vi "Tray_TraySetPanel.vi"(8 "error in":errorcluster, 11 "Enum_TrayType":T1) -> (0 "error Out":errorcluster)   [LabVIEW 2015]
uses:
  subvi/Tray/Tray_TrayName.ctl
  <vilib>/Utility/miscctls.llb/LVPointTypeDef.ctl
  subvi/Tray/Tray_TrayCtrl_Action.ctl
  LLB/Message/Ctrl/MsgDataInput.ctl
  LLB/Message/Ctrl/MsgPageSelect.ctl
  LLB/Message/Ctrl/MsgTyp.ctl
  LLB/Message/Ctrl/LogType.ctl
  global/Tray_ArrAndData.vi
  LLB/Message/MsgShowAndLog.lvlib
panel:
  out "Flg_Edit":bool
  out "TrayItemStatus":bool[][](array[boolean])
  out "Tray":cluster{"X":i32, "Y":i32}
  in  "Btn_Ini":bool
  in  "Set":bool
  in  "ItemExist":u32(colorbox)=16860
  in  "NoItem":u32(colorbox)=11121611
  in  "SingleSet":bool caption="SetType"
  in  "StatusArr":bool[][](array[boolean])
  in  "Stop Button":bool
  in  "BtnArr":bool[][](array[boolean])
  out "TrayIn":cluster{"Color":u32[][], "Data":string[][]}={"Color"=[[16860, 16860, 16860, 16860, 16860, 16860, 16860, 16860], [16860, 16860, 16860, 16860, 16860, 16860, 16860, 16860], [16860, 16860, 16860, 16860, 16860, 16860, 16860, 16860], [16860, 16860, 16860, 16860, 16860, 16860, 16860, 16860], [16860, 16860, 16860, 16860, 16860, 16860, 16860, 16860], [16860, 16860, 16860, 16860, 16860, 16860, 16860, 16860], [16860, 16860, 16860, 16860, 16860, 16860, 16860, 16860], [16860, 16860, 16860, 16860, 16860, 16860, 16860, 16860], [16860, 16860, 16860, 16860, 16860, 16860, 16860, 16860], [16860, 16860, 16860, 16860, 16860, 16860, 16860, 16860], [16860, 16860, 16860, 16860, 16860, 16860, 16860, 16860], [16860, 16860, 16860, 16860, 16860, 16860, 16860, 16860]], "Data"=[["", "", "", "", "", "", "", ""], ["", "", "", "", "", "", "", ""], ["", "", "", "", "", "", "", ""], ["", "", "", "", "", "", "", ""], ["", "", "", "", "", "", "", ""], ["", "", "", "", "", "", "", ""], ["", "", "", "", "", "", "", ""], ["", "", "", "", "", "", "", ""], ["", "", "", "", "", "", "", ""], ["", "", "", "", "", "", "", ""], ["", "", "", "", "", "", "", ""], ["", "", "", "", "", "", "", ""]]}
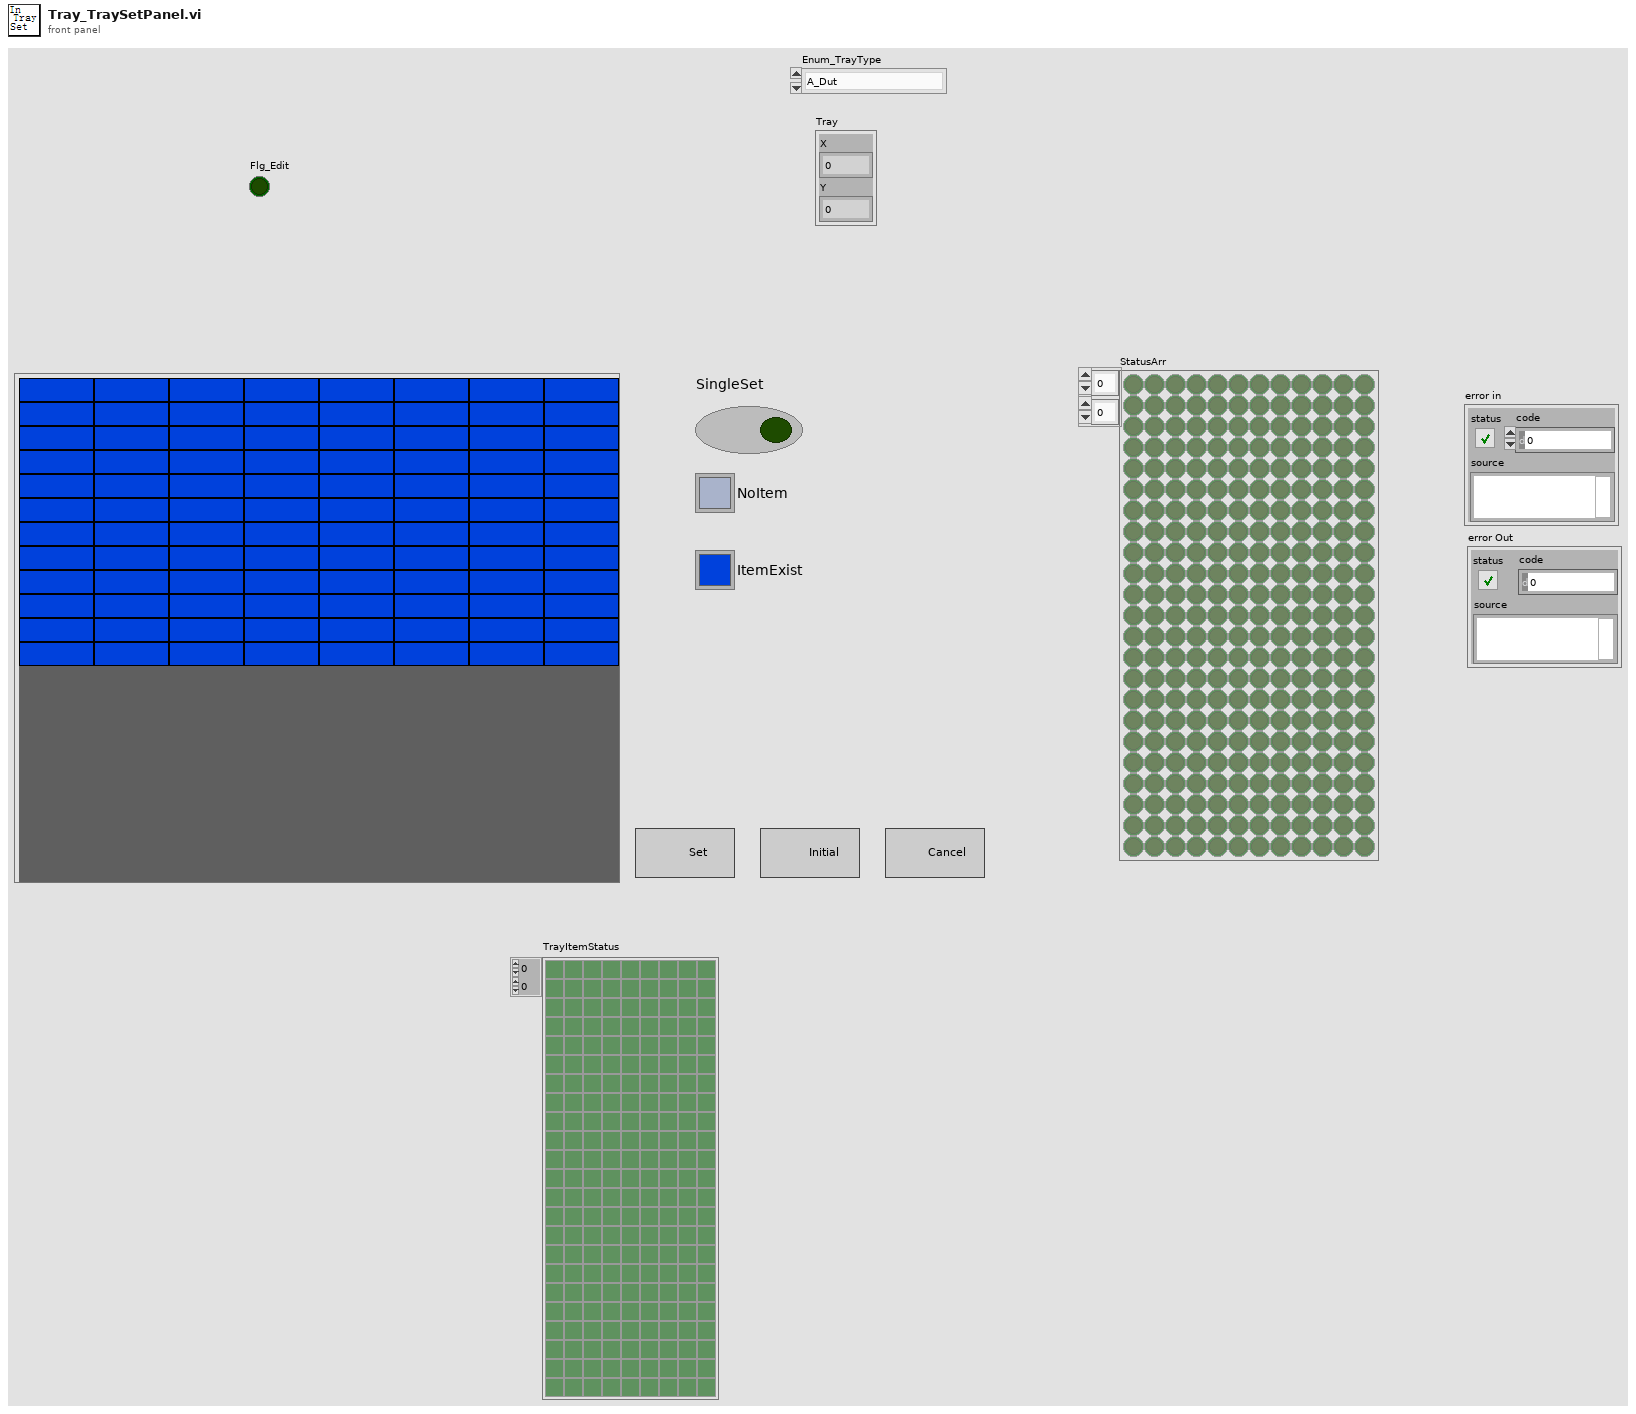
[diagram p1: front panel]
types:
  T1 = typedef "Tray_TrayName.ctl" = enum16{"A_Dut", "B_Pass", "C_NGR", "D_NGL"}
  T2 = typedef "LVPointTypeDef.ctl" = cluster{"Horizontal":i16, "Vertical":i16}
  T3 = cluster{"BtnArr":refnum<vi>, "BtnRef":refnum<vi>}
  T4 = typedef "MsgDataInput.ctl" = cluster{"MsgPageSelect":T5, "Type":T6, "LogType":T7, "Msg":string, "Time":string}
  T5 = typedef "MsgShowAndLog.lvlib/MsgPageSelect.ctl" = enum16{"System", "Robot", "IO", "CCD", "Action", "Alarm", "ATS"}
  T6 = typedef "MsgShowAndLog.lvlib/MsgTyp.ctl" = enum16{"SYS", "TCP/IP", "IO", "CCD", "Action", "RS232"}
  T7 = typedef "MsgShowAndLog.lvlib/LogType.ctl" = enum16{"AutoRun", "Manual", "Error", "ATS"}
  T8 = typedef "Tray_TrayCtrl_Action.ctl" = enum16{"InitialTray", "TrayOut", "TrayIn", "SetTray", "TrayDataToUI"}
  T9 = cluster{"XY_ATray":cluster{"X":i32, "Y":i32}, "Initial color":u32, "FinalColor":u32}
  T10 = cluster{"XY_BTray":cluster{"X":i32, "Y":i32}, "Initial color":u32, "FinalColor":u32}
  T11 = cluster{"XY_CTray":cluster{"X":i32, "Y":i32}, "Initial color":u32, "FinalColor":u32}
  T12 = cluster{"XY_DTray":cluster{"X":i32, "Y":i32}, "Initial color":u32, "FinalColor":u32}
  T13 = typedef "LVPositionTypeDef.ctl" = cluster{"Left":i32, "Top":i32}
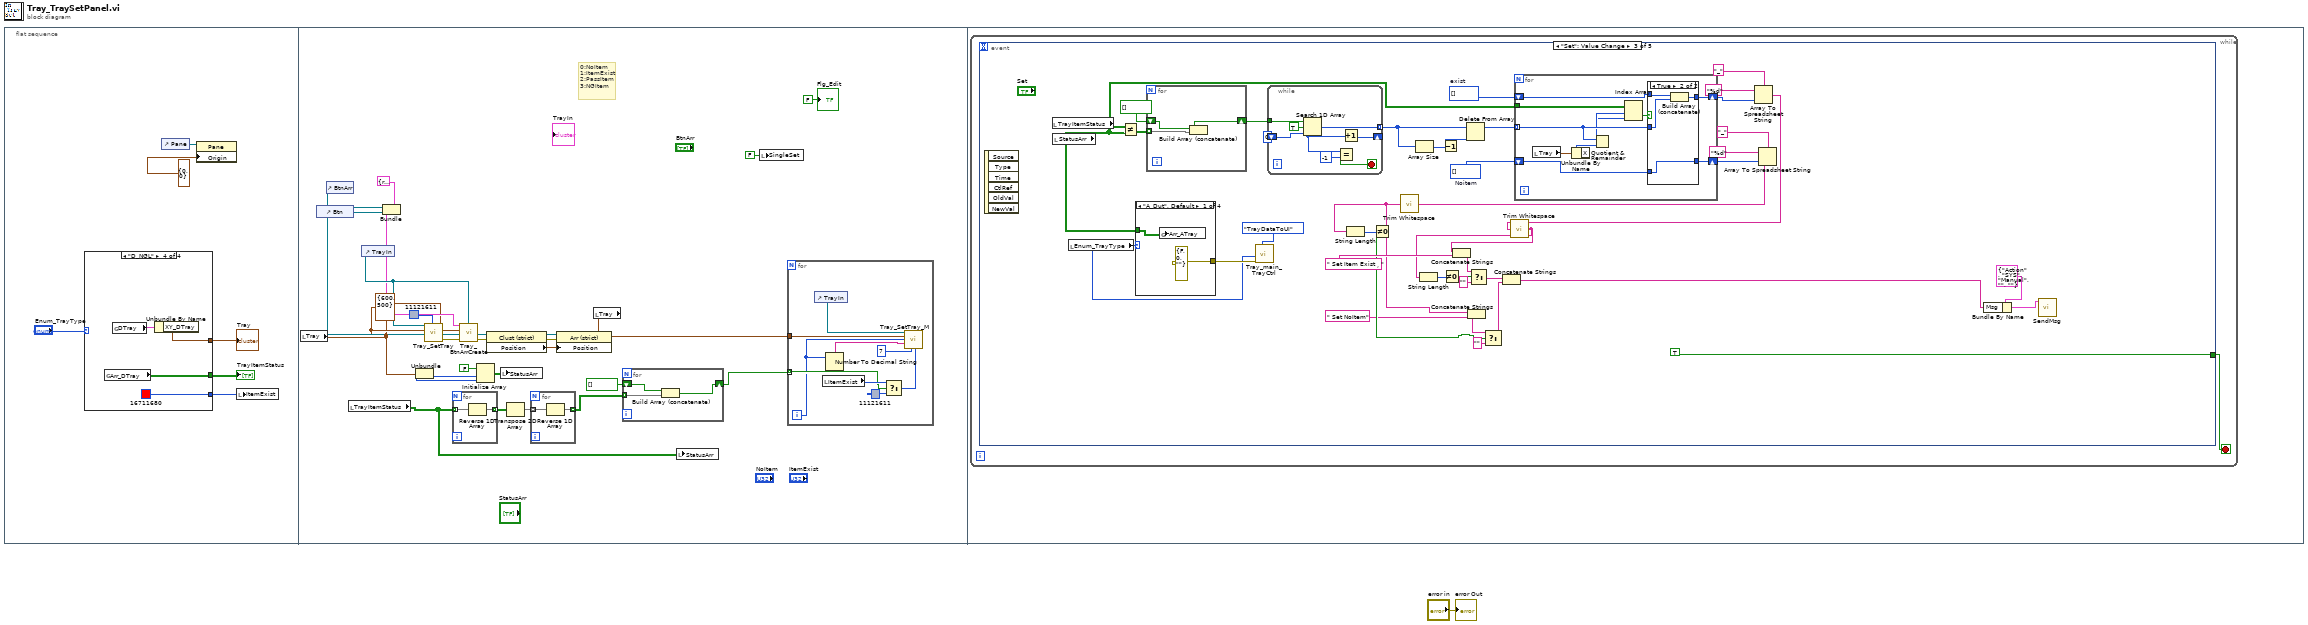
[diagram p0: block diagram]
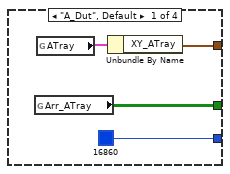
[diagram p2: hidden frame]
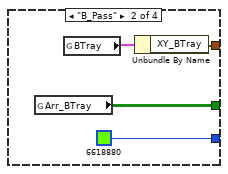
[diagram p3: hidden frame]
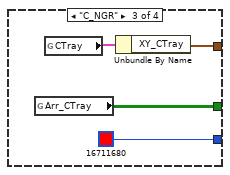
[diagram p4: hidden frame]
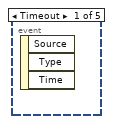
[diagram p5: hidden frame]
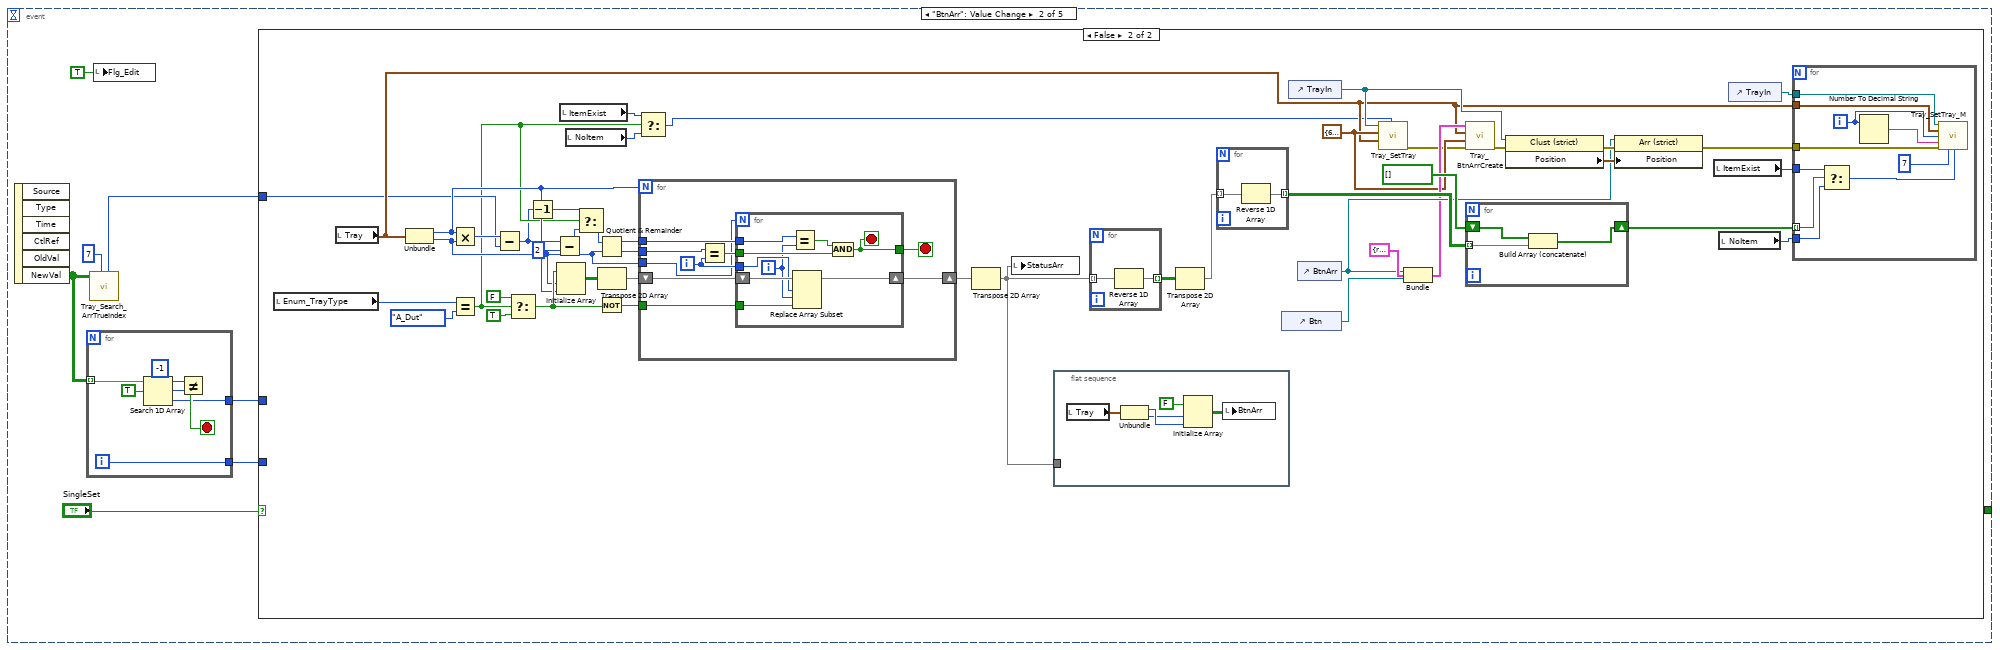
[diagram p6: hidden frame]
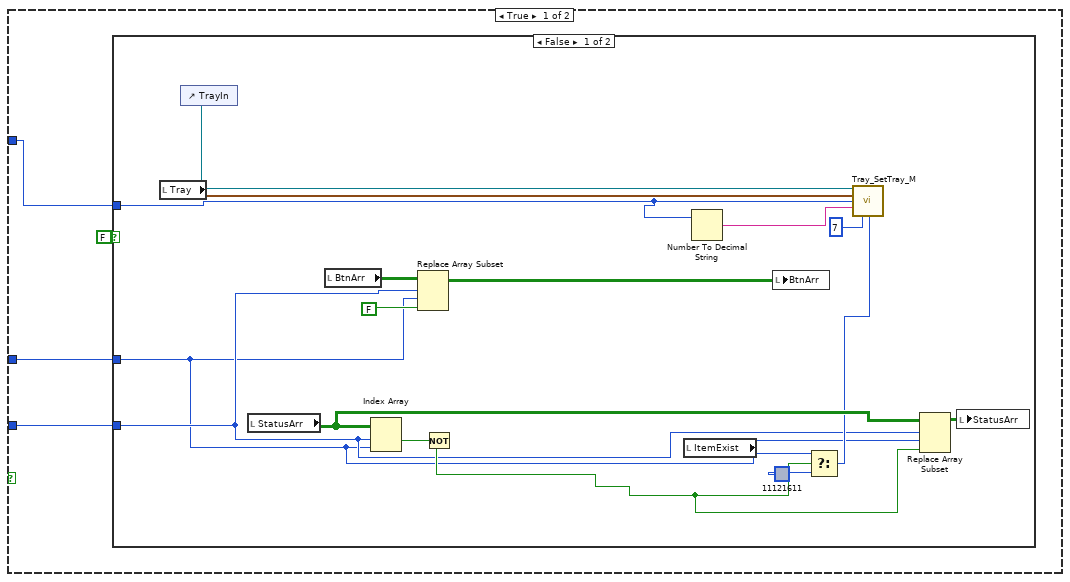
[diagram p7: hidden frame]
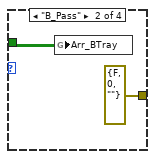
[diagram p9: hidden frame]
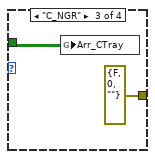
[diagram p10: hidden frame]
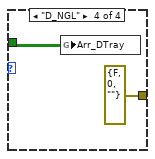
[diagram p11: hidden frame]
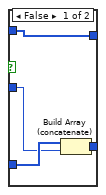
[diagram p12: hidden frame]
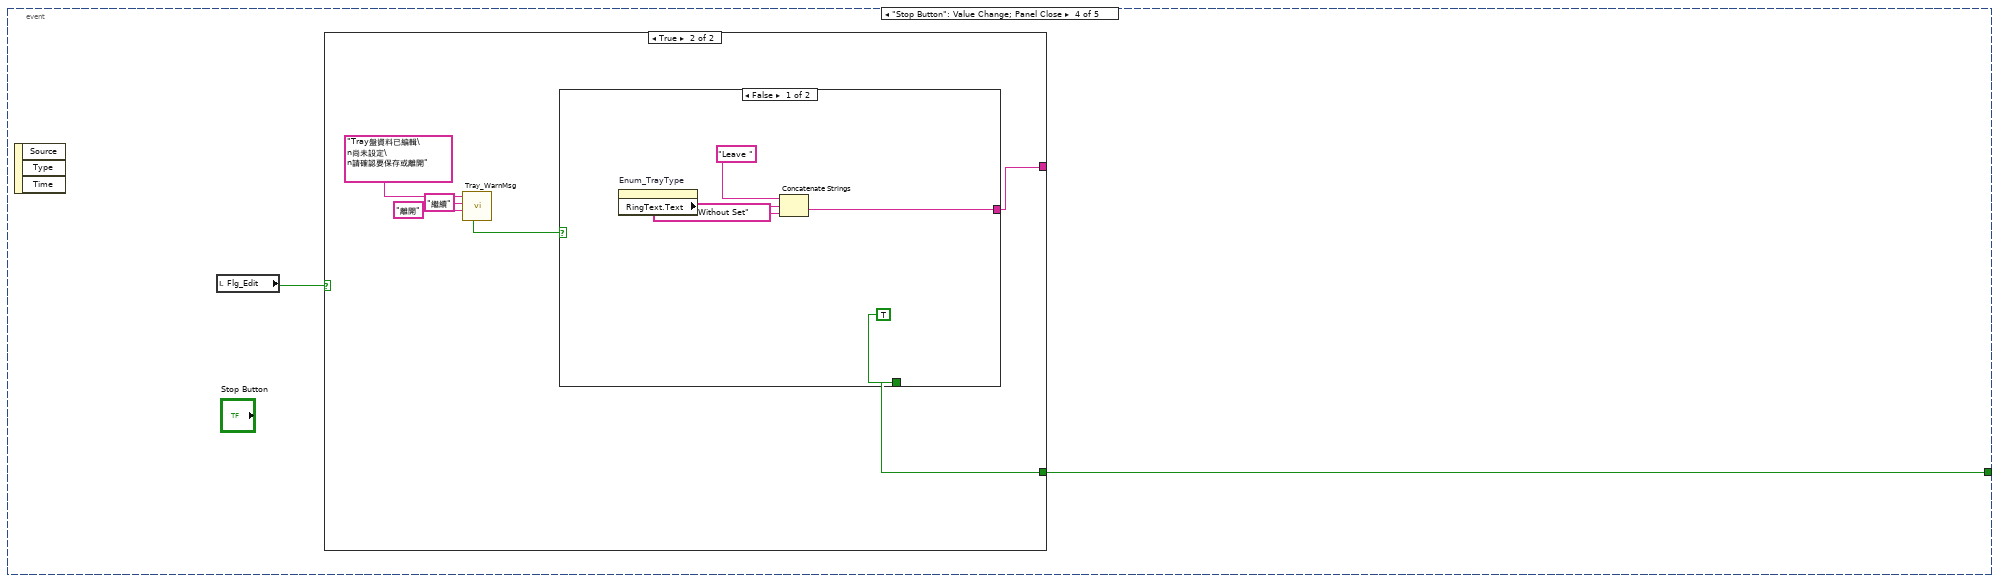
[diagram p13: hidden frame]
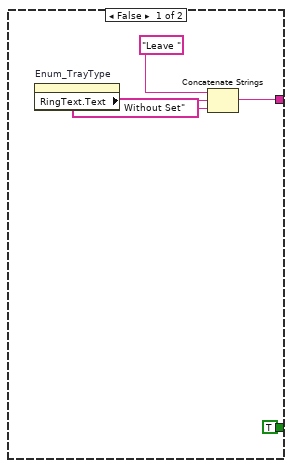
[diagram p14: hidden frame]
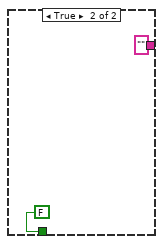
[diagram p15: hidden frame]
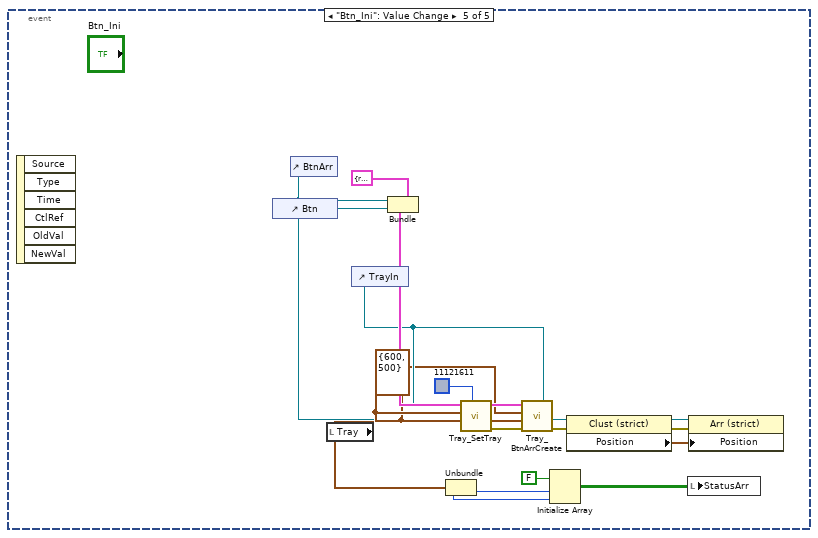
[diagram p16: hidden frame]
diagram:
  n1 = flat-sequence {
    frame #0 {
      n2 = case shown="\"D_NGL\"" "Enum_TrayType" {
        tunnel: [w8 w12 w16 w20] -> w2
        tunnel: [u32 16860 ("ItemExist") u32 6618880 ("ItemExist") u32 16711680 ("ItemExist") u32 16711680 ("ItemExist")] -> w5
        tunnel: [w10 w14 w18 w22] -> w4
        frame "A_Dut", Default {
          n3 = global read "Tray_ArrAndData.vi" "Arr_ATray"() -> (w10:bool[][])
          n4 = global read "Tray_ArrAndData.vi" "ATray"() -> (w9:T9)
          n5 = Unbundle By Name(w9) -> ("XY_ATray"=w8:cluster{"X":i32, "Y":i32})
        }
        frame "B_Pass" {
          n6 = global read "Tray_ArrAndData.vi" "Arr_BTray"() -> (w14:bool[][])
          n7 = global read "Tray_ArrAndData.vi" "BTray"() -> (w13:T10)
          n8 = Unbundle By Name(w13) -> ("XY_BTray"=w12:cluster{"X":i32, "Y":i32})
        }
        frame "C_NGR" {
          n9 = global read "Tray_ArrAndData.vi" "Arr_CTray"() -> (w18:bool[][])
          n10 = global read "Tray_ArrAndData.vi" "CTray"() -> (w17:T11)
          n11 = Unbundle By Name(w17) -> ("XY_CTray"=w16:cluster{"X":i32, "Y":i32})
        }
        frame "D_NGL" {
          n12 = global read "Tray_ArrAndData.vi" "Arr_DTray"() -> (w22:bool[][])
          n13 = global read "Tray_ArrAndData.vi" "DTray"() -> (w21:T12)
          n14 = Unbundle By Name(w21) -> ("XY_DTray"=w20:cluster{"X":i32, "Y":i32})
        }
      }
      "Tray" <- w2
      "TrayItemStatus" <- w4
      n15 = control-ref of="Pane"() -> (w6:refnum<vi>)
      n16 = property class="Pane"(reference=w6, "Origin"=T2 {"Horizontal"=0, "Vertical"=0}) -> ()  [unwired: 1 in, 2 out]
      n17 = local write "ItemExist"(w5) -> ()
    }
    frame #1 {
      w36 = cluster{"x":u32, "y":u32} {"x"=600, "y"=500} ("MaxArea")
      # "0:NoItem\n1:ItemExist\n2:PassItem\n3:NGItem"
      n18 = local read "Tray"() -> (w32:cluster{"X":i32, "Y":i32})
      n19 = control-ref of="Btn"() -> (w45:refnum<vi>)
      n20 = control-ref of="BtnArr"() -> (w42:refnum<vi>)
      n21 = local read "TrayItemStatus"() -> (w27:bool[][])
      n22 = control-ref of="TrayIn"() -> (w47:refnum<vi>)
      n23 = Bundle(cluster=T3 {"BtnArr"=refnum, "BtnRef"=refnum} ("Refin"), "BtnArr"=w42, "BtnRef"=w45) -> (w41:T3)
      n24 = Unbundle(w32) -> ("X"=w37:i32, "Y"=w38:i32)
      n25 = call "Tray_SetTray.vi"("Initial color"=u32 11121611, "GridSize"=w32, "MaxArea"=w36, "Tray in"=w47) -> ("error out"=w35:errorcluster)  [unwired: 7 in]
      n26 = for {
        tunnel: w27 -> [w53] mode=indexing
        tunnel: [w52] -> w29 mode=indexing
        n27 = Reverse 1D Array(array=w53) -> (reversed array=w52:bool[])
      }
      n28 = call "Tray_BtnArrCreate.vi"("error in"=w35, "MaxArea"=w36, "GridSize"=w32, "Refin"=w41) -> ("error out"=w34:errorcluster)  [unwired: 7 in]
      n29 = Initialize Array(FALSE, w38, w37) -> (w40:bool[][])
      n30 = property class="Clust (strict)"(reference=w47, error in=w34) -> (error out=w44:errorcluster, "Position"=w46:T13)  [unwired: 1 out]
      n31 = local write "StatusArr"(w40) -> ()
      n32 = Transpose 2D Array(2D array=w29) -> (transposed array=w28:bool[][])
      n33 = for {
        tunnel: w28 -> [w55] mode=indexing
        tunnel: [w54] -> w26 mode=indexing
        n34 = Reverse 1D Array(array=w55) -> (reversed array=w54:bool[])
      }
      n35 = property class="Arr (strict)"(reference=w42, error in=w44, "Position"=w46) -> ()  [unwired: 2 out]
      n36 = local read "Tray"() -> (w31:cluster{"X":i32, "Y":i32})
      n37 = for {
        shift-right: [w49] -> w25
        shift-left: bool[] [] -> [w51]
        tunnel: w26 -> [w50] mode=indexing
        n38 = Build Array (concatenate)(w51, w50) -> (w49:bool[])
      }
      n39 = local write "StatusArr"(w27) -> ()
      n40 = local write "SingleSet"(FALSE ("SingleSet")) -> ()
      n41 = for {
        tunnel: w31 -> [w64]
        tunnel: w25 -> [w58] mode=indexing
        i -> [w57]
        n42 = control-ref of="TrayIn"() -> (w60:refnum<vi>)
        n43 = local read "ItemExist"() -> (w63:u32)
        n44 = Number To Decimal String(number=w57) -> (decimal integer string=w56:string)  [unwired: 1 in]
        n45 = Select(t=w63, s=w58, f=u32 11121611 ("Initial color")) -> (s? t:f=w62:u32)
        n46 = call "Tray_SetTray_M.vi"("TrayIn"=w60, "GridSize"=w64, "Index Number"=w57, "String"=w56, "Direction"=u16 7, "Color Box"=w62) -> ()  [unwired: 9 in, 1 out]
      }
      "Flg_Edit" <- FALSE ("Flg_Edit")
    }
    frame #2 {
      n47 = while {
        stop <- w65 stop-if-true
        n48 = event shown="[2] \"Set\": Value Change" {
          selector: _ -> [_ _ _ _ _]
          dyn-events: _ -> [_ _ _ _ _]
          timeout: _ -> [_ _ _ _ _]
          tunnel: [_ _ TRUE w263 _] -> w65
          event Timeout {
            n49 = event-data() -> ()  [unwired: 1 in, 3 out]
          }
          event "BtnArr": Value Change {
            n50 = event-data() -> ("NewVal"=w68:bool[][])  [unwired: 1 in, 5 out]
            n51 = for {
              tunnel: w68 -> [w78] mode=indexing
              tunnel: [w74] -> w67
              tunnel: [w73] -> w66
              i -> [w73]
              stop <- w75 stop-if-true
              n52 = Search 1D Array(1D array=w78, element=TRUE) -> (index of element=w74:i32)  [unwired: 1 in]
              n53 = Not Equal?(x=-1, y=w74) -> (x != y?=w75:bool)
            }
            n54 = call "Tray_Search_ArrTrueIndex.vi"("Direction"=u16 7, "Input_Arr"=w68) -> ("SearchTrueIndex"=w70:i32)  [unwired: 7 in, 2 out]
            n55 = local write "Flg_Edit"(TRUE ("Flg_Edit")) -> ()
            n56 = case shown="False" "SingleSet" {
              tunnel: w70 -> [w80 w106]
              tunnel: w67 -> [w82 _]
              tunnel: w66 -> [w81 _]
              frame True {
                n57 = case shown="False" FALSE {
                  tunnel: w82 -> [w85 _]
                  tunnel: w81 -> [w86 _]
                  tunnel: w80 -> [w84 _]
                  frame False {
                    n58 = local read "Tray"() -> (w88:cluster{"X":i32, "Y":i32})
                    n59 = control-ref of="TrayIn"() -> (w99:refnum<vi>)
                    n60 = local read "StatusArr"() -> (w94:bool[][])
                    n61 = local read "BtnArr"() -> (w98:bool[][])
                    n62 = Index Array(array=w94, index (row)=w86, index (col)=w85) -> (element=w90:bool)
                    n63 = Replace Array Subset(array=w98, new element=FALSE ("new element/subarray"), index (row)=w86, index (col)=w85) -> (w97:bool[][])
                    n64 = Not(x=w90) -> (.not. x?=w89:bool)
                    n65 = local read "ItemExist"() -> (w91:u32)
                    n66 = Number To Decimal String(number=w84) -> (decimal integer string=w83:string)  [unwired: 1 in]
                    n67 = local write "BtnArr"(w97) -> ()
                    n68 = Select(t=w91, s=w89, f=u32 11121611 ("Initial color")) -> (s? t:f=w93:u32)
                    n69 = call "Tray_SetTray_M.vi"("TrayIn"=w99, "GridSize"=w88, "Index Number"=w84, "String"=w83, "Direction"=u16 7, "Color Box"=w93) -> ()  [unwired: 9 in, 1 out]
                    n70 = Replace Array Subset(array=w94, new element=w89, index (row)=w86, index (col)=w85) -> (w92:bool[][])
                    n71 = local write "StatusArr"(w92) -> ()
                  }
                  frame True {
                  }
                }
              }
              frame False {
                w125 = cluster{"x":u32, "y":u32} {"x"=600, "y"=500} ("MaxArea")
                n72 = local read "Enum_TrayType"() -> (w134:T1)
                n73 = local read "Tray"() -> (w120:cluster{"X":i32, "Y":i32})
                n74 = Unbundle(w120) -> ("X"=w109:i32, "Y"=w110:i32)
                n75 = Multiply(x=w109, y=w110) -> (x*y=w117:i32)
                n76 = Equal?(x=w134, y=Tray_TrayName."A_Dut") -> (x = y?=w104:bool)
                n77 = Subtract(x=w117, y=w106) -> (x-y=w101:i32)
                n78 = Select(t=FALSE, s=w104, f=TRUE) -> (s? t:f=w116:bool)
                n79 = Decrement(x=w101) -> (x-1=w103:i32)
                n80 = Subtract(x=w101, y=2) -> (x-y=w102:i32)
                n81 = Initialize Array(w116, w110, w109) -> (w115:bool[][])
                n82 = local read "ItemExist"() -> (w143:u32)
                n83 = local read "NoItem"() -> (w144:u32)
                n84 = Select(t=w103, s=w104, f=w102) -> (s? t:f=w105:i32)
                n85 = Not(x=w116) -> (.not. x?=w111:bool)
                n86 = Quotient & Remainder(x=w105, y=w110) -> (x-y*floor(x/y)=w108:i32, floor(x/y)=w112:i32)
                n87 = Transpose 2D Array(2D array=w115) -> (transposed array=w114:bool[][])
                n88 = Select(t=w143, s=w104, f=w144) -> (s? t:f=w107:u32)
                n89 = for {
                  N: w109 -> [_]
                  shift-right: [w164] -> w113
                  shift-left: w114 -> [w165]
                  tunnel: w108 -> [w163]
                  tunnel: w112 -> [w162]
                  tunnel: w111 -> [w158]
                  tunnel: w110 -> [w157]
                  i -> [w159]
                  stop <- w160 stop-if-true
                  n90 = Equal?(x=w162, y=w159) -> (x = y?=w161:bool)
                  n91 = for {
                    N: w157 -> [_]
                    shift-right: [w173] -> w164
                    shift-left: w165 -> [w174]
                    tunnel: w163 -> [w172]
                    tunnel: w161 -> [w170]
                    tunnel: [w169] -> w160
                    tunnel: w159 -> [w168]
                    tunnel: w158 -> [w166]
                    i -> [w167]
                    stop <- w169 stop-if-true
                    n92 = Equal?(x=w172, y=w167) -> (x = y?=w171:bool)
                    n93 = Replace Array Subset(array=w174, new element=w166, index (row)=w168, index (col)=w167) -> (w173:bool[][])
                    n94 = And(x=w171, y=w170) -> (x .and. y?=w169:bool)
                  }
                }
                n95 = Transpose 2D Array(2D array=w113) -> (transposed array=w137:bool[][])
                n96 = local write "StatusArr"(w137) -> ()
                n97 = flat-sequence {
                  tunnel: w137 -> [_]
                  frame #0 {
                    n98 = local read "Tray"() -> (w152:cluster{"X":i32, "Y":i32})
                    n99 = Unbundle(w152) -> ("X"=w155:i32, "Y"=w154:i32)
                    n100 = Initialize Array(FALSE, w154, w155) -> (w153:bool[][])
                    n101 = local write "BtnArr"(w153) -> ()
                  }
                }
                n102 = for {
                  tunnel: w137 -> [w149] mode=indexing
                  tunnel: [w148] -> w135 mode=indexing
                  n103 = Reverse 1D Array(array=w149) -> (reversed array=w148:bool[])
                }
                n104 = Transpose 2D Array(2D array=w135) -> (transposed array=w136:bool[][])
                n105 = for {
                  tunnel: w136 -> [w151] mode=indexing
                  tunnel: [w150] -> w139 mode=indexing
                  n106 = Reverse 1D Array(array=w151) -> (reversed array=w150:bool[])
                }
                n107 = control-ref of="Btn"() -> (w130:refnum<vi>)
                n108 = control-ref of="TrayIn"() -> (w132:refnum<vi>)
                n109 = control-ref of="BtnArr"() -> (w127:refnum<vi>)
                n110 = call "Tray_SetTray.vi"("Initial color"=w107, "GridSize"=w120, "MaxArea"=w125, "Tray in"=w132) -> ("error out"=w124:errorcluster)  [unwired: 7 in]
                n111 = Bundle(cluster=T3 {"BtnArr"=refnum, "BtnRef"=refnum} ("Refin"), "BtnArr"=w127, "BtnRef"=w130) -> (w126:T3)
                n112 = call "Tray_BtnArrCreate.vi"("error in"=w124, "MaxArea"=w125, "GridSize"=w120, "Refin"=w126) -> ("error out"=w123:errorcluster)  [unwired: 7 in]
                n113 = for {
                  shift-right: [w145] -> w140
                  shift-left: bool[] [] -> [w147]
                  tunnel: w139 -> [w146] mode=indexing
                  n114 = Build Array (concatenate)(w147, w146) -> (w145:bool[])
                }
                n115 = property class="Clust (strict)"(reference=w132, error in=w123) -> (error out=w129:errorcluster, "Position"=w131:T13)  [unwired: 1 out]
                n116 = property class="Arr (strict)"(reference=w127, error in=w129, "Position"=w131) -> (error out=w122:errorcluster)  [unwired: 1 out]
                n117 = local read "ItemExist"() -> (w141:u32)
                n118 = local read "NoItem"() -> (w142:u32)
                n119 = control-ref of="TrayIn"() -> (w121:refnum<vi>)
                n120 = for {
                  tunnel: w122 -> [w184]
                  tunnel: w121 -> [w183]
                  tunnel: w120 -> [w182]
                  tunnel: w140 -> [w178] mode=indexing
                  tunnel: w141 -> [w177]
                  tunnel: w142 -> [w176]
                  i -> [w180]
                  n121 = Select(t=w177, s=w178, f=w176) -> (s? t:f=w175:u32)
                  n122 = Number To Decimal String(number=w180) -> (decimal integer string=w179:string)  [unwired: 1 in]
                  n123 = call "Tray_SetTray_M.vi"("TrayIn"=w183, "GridSize"=w182, "Index Number"=w180, "String"=w179, "error in"=w184, "Direction"=u16 7, "Color Box"=w175) -> ()  [unwired: 8 in, 1 out]
                }
              }
            }
          }
          event "Set": Value Change {
            w215 = i32[] []  # Noitem
            w216 = i32[] []  # exist
            n124 = event-data() -> ()  [unwired: 1 in, 6 out]
            n125 = local read "TrayItemStatus"() -> (w224:bool[][])
            n126 = local read "StatusArr"() -> (w208:bool[][])
            n127 = local read "Enum_TrayType"() -> (w188:T1)
            n128 = Not Equal?(x=w224, y=w208) -> (x != y?=w223:bool[][])
            n129 = case shown="\"A_Dut\", Default" w188 {
              tunnel: w208 -> [w226 w228 w230 w232]
              tunnel: [errorcluster {"status"=FALSE, "code"=0, "source"=""} ("error constant") errorcluster {"status"=FALSE, "code"=0, "source"=""} ("error constant") errorcluster {"status"=FALSE, "code"=0, "source"=""} ("error constant") errorcluster {"status"=FALSE, "code"=0, "source"=""} ("error constant")] -> w206
              frame "A_Dut", Default {
                n130 = global write "Tray_ArrAndData.vi" "Arr_ATray"(w226) -> ()
              }
              frame "B_Pass" {
                n131 = global write "Tray_ArrAndData.vi" "Arr_BTray"(w228) -> ()
              }
              frame "C_NGR" {
                n132 = global write "Tray_ArrAndData.vi" "Arr_CTray"(w230) -> ()
              }
              frame "D_NGL" {
                n133 = global write "Tray_ArrAndData.vi" "Arr_DTray"(w232) -> ()
              }
            }
            n134 = for {
              tunnel: w223 -> [w255] mode=indexing
              shift-right: [w254] -> w221
              shift-left: bool[] [] -> [w253]
              n135 = Build Array (concatenate)(w253, w255) -> (w254:bool[])
            }
            n136 = call "Tray_main_TrayCtrl.vi"("Enum"=Tray_TrayCtrl_Action."TrayDataToUI", "error in"=w206, "TrayType"=w188) -> ()  [unwired: 8 in, 1 out]
            n137 = while {
              tunnel: w221 -> [w262]
              shift-right: [w259] -> _
              shift-left: 0 ("index of element") -> [w260]
              tunnel: [w258] -> w219 mode=indexing
              stop <- w256 stop-if-true
              n138 = Search 1D Array(1D array=w262, element=TRUE, start index (0)=w260) -> (index of element=w258:i32)
              n139 = Equal?(x=w258, y=-1) -> (x = y?=w256:bool)
              n140 = Increment(x=w258) -> (x+1=w259:i32)
            }
            n141 = Array Size(array=w219) -> (size(s)=w218:i32)
            n142 = Decrement(x=w218) -> (x-1=w217:i32)
            n143 = Delete From Array(array=w219, index=w217) -> (array with subset deleted=w205:i32[])  [unwired: 1 in, 1 out]
            n144 = for {
              tunnel: w205 -> [w239] mode=indexing
              tunnel: w208 -> [w244]
              shift-right: [w238] -> w212
              shift-left: w216 -> [w240]
              shift-right: [w236] -> w204
              shift-left: w215 -> [w237]
              n145 = local read "Tray"() -> (w243:cluster{"X":i32, "Y":i32})
              n146 = Unbundle By Name(w243) -> ("X"=w242:i32)
              n147 = Quotient & Remainder(x=w239, y=w242) -> (x-y*floor(x/y)=w234:i32, floor(x/y)=w235:i32)
              n148 = Index Array(array=w244, index (row)=w235, index (col)=w234) -> (element=w241:bool)
              n149 = case shown="True" w241 {
                tunnel: w240 -> [w248 w252]
                tunnel: w239 -> [w246 w251]
                tunnel: [w248 w250] -> w238
                tunnel: w237 -> [w247 w249]
                tunnel: [w245 w249] -> w236
                frame False {
                  n150 = Build Array (concatenate)(w247, w246) -> (w245:i32[])
                }
                frame True {
                  n151 = Build Array (concatenate)(w252, w251) -> (w250:i32[])
                }
              }
            }
            n152 = Array To Spreadsheet String(delimiter (Tab)="_", array=w212, 3:"%d" ("format string")) -> (spreadsheet string=w190:string)
            n153 = call <vilib>:"Trim Whitespace.vi"("string"=w190) -> ("trimmed string"=w189:string)  [unwired: 1 in]
            n154 = String Length(string=w189) -> (length=w203:i32)
            n155 = Not Equal To 0?(x=w203) -> (x != 0?=w201:bool)
            n156 = Concatenate Strings(w189, " Set Item Exist，" ("string")) -> (w199:string)
            n157 = Select(t=w199, s=w201, f="") -> (s? t:f=w192:string)
            n158 = Array To Spreadsheet String(delimiter (Tab)="_", array=w204, 3:"%d" ("format string")) -> (spreadsheet string=w209:string)
            n159 = call <vilib>:"Trim Whitespace.vi"("string"=w209) -> ("trimmed string"=w194:string)  [unwired: 1 in]
            n160 = String Length(string=w194) -> (length=w202:i32)
            n161 = Not Equal To 0?(x=w202) -> (x != 0?=w195:bool)
            n162 = Concatenate Strings(w194, " Set NoItem" ("string")) -> (w196:string)
            n163 = Select(t=w196, s=w195, f="") -> (s? t:f=w191:string)
            n164 = Concatenate Strings(w192, w191) -> (w185:string)
            n165 = Bundle By Name(cluster=T4 {"MsgPageSelect"=enum."Action", "Type"=enum."SYS", "LogType"=enum."Manual", "Msg"="", "Time"=""} ("DataIn"), "Msg"=w185) -> (w186:T4)
            n166 = call "SendMsg.vi"("DataIn"=w186) -> ()  [unwired: 10 in, 1 out]
          }
          event "Stop Button": Value Change; Panel Close {
            n167 = event-data() -> ()  [unwired: 1 in, 3 out]
            n168 = local read "Flg_Edit"() -> (w264:bool)
            n169 = case shown="True" w264 {
              tunnel: [w266 w271] -> _
              tunnel: [TRUE ("Stop Button") w270] -> w263
              frame False {
                n170 = property on="Enum_TrayType" class="Enum (strict)"() -> ("RingText.Text"=w268:string)  [unwired: 2 in, 2 out]
                n171 = Concatenate Strings("Leave ", w268, "SetPanel Without Set" ("string")) -> (w266:string)
              }
              frame True {
                n172 = call "Tray_WarnMsg.vi"("Boolean Text Cancel"="離開", "Boolean Text OK"="繼續", "Msg"="Tray盤資料已編輯\n尚未設定\n請確認要保存或離開") -> ("OK?"=w272:bool)  [unwired: 8 in]
                n173 = case shown="False" w272 {
                  tunnel: [w277 ""] -> w271
                  tunnel: [TRUE ("Stop Button") FALSE ("Stop Button")] -> w270
                  frame False {
                    n174 = property on="Enum_TrayType" class="Enum (strict)"() -> ("RingText.Text"=w279:string)  [unwired: 2 in, 2 out]
                    n175 = Concatenate Strings("Leave ", w279, "SetPanel Without Set" ("string")) -> (w277:string)
                  }
                  frame True {
                  }
                }
              }
            }
          }
          event "Btn_Ini": Value Change {
            w296 = cluster{"x":u32, "y":u32} {"x"=600, "y"=500} ("MaxArea")
            n176 = event-data() -> ()  [unwired: 1 in, 6 out]
            n177 = control-ref of="Btn"() -> (w287:refnum<vi>)
            n178 = control-ref of="BtnArr"() -> (w290:refnum<vi>)
            n179 = local read "Tray"() -> (w283:cluster{"X":i32, "Y":i32})
            n180 = control-ref of="TrayIn"() -> (w285:refnum<vi>)
            n181 = Bundle(cluster=T3 {"BtnArr"=refnum, "BtnRef"=refnum} ("Refin"), "BtnArr"=w290, "BtnRef"=w287) -> (w291:T3)
            n182 = Unbundle(w283) -> ("X"=w295:i32, "Y"=w294:i32)
            n183 = call "Tray_SetTray.vi"("Initial color"=u32 11121611, "GridSize"=w283, "MaxArea"=w296, "Tray in"=w285) -> ("error out"=w297:errorcluster)  [unwired: 7 in]
            n184 = call "Tray_BtnArrCreate.vi"("error in"=w297, "MaxArea"=w296, "GridSize"=w283, "Refin"=w291) -> ("error out"=w298:errorcluster)  [unwired: 7 in]
            n185 = Initialize Array(FALSE, w294, w295) -> (w292:bool[][])
            n186 = property class="Clust (strict)"(reference=w285, error in=w298) -> (error out=w288:errorcluster, "Position"=w286:T13)  [unwired: 1 out]
            n187 = local write "StatusArr"(w292) -> ()
            n188 = property class="Arr (strict)"(reference=w290, error in=w288, "Position"=w286) -> ()  [unwired: 2 out]
          }
        }
      }
    }
  }
  "error Out" <- "error in"
